vi "MassData Parameter Support Demo.vi"() -> ()   [LabVIEW 2017]
uses:
  MassData-Parameter/_support/Operation-FGV-MassData.ctl
  b1bc9acf-e850-46c1-b3cf-cc66e9187574.vi
  537af5e7-dcec-4c12-9422-676432e19088.vi
  MassData-Parameter/CSM MassData Parameter Support.lvlib
panel:
  in  "stop":bool
  out "Thermometer":cluster{dbl, dbl}(slide)={0.0, 6224.489795918367} scale=0.0..1000000.0 scale format="%#_6p"
  out "Argument":string
  out "Waveform Graph":i32[](graph)
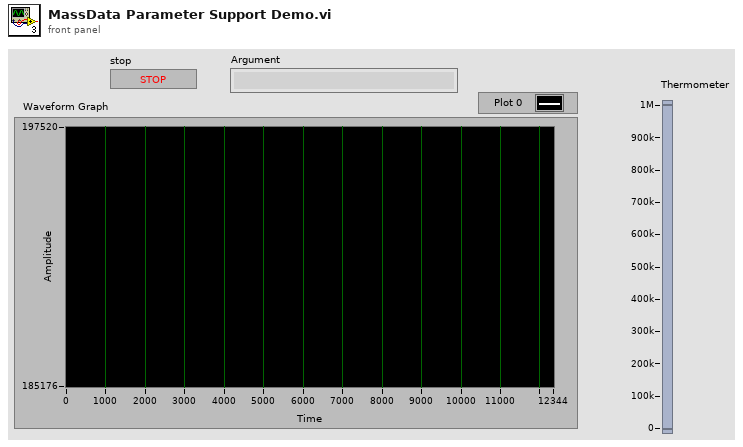
[diagram p1: front panel]
types:
  T1 = typedef "CSM MassData Parameter Support.lvlib/Operation-FGV-MassData.ctl" = enum16{"Initialize", "Read", "Write", "Status", "Release"}
  T2 = typedef "CSM MassData Parameter Support.lvlib/Def-MassDataOper-Status.ctl" = cluster{"Start":i32, "Size":i32, "Total":i32}
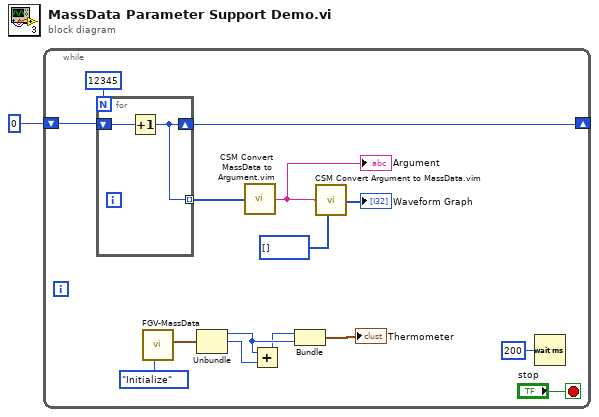
[diagram p0: block diagram]
diagram:
  n1 = while {
    shift-right: [w4] -> _
    shift-left: 0 -> [w5]
    stop <- "stop" stop-if-true
    n2 = for {
      N: 12345 -> [_]
      tunnel: [w17] -> w15 mode=indexing
      shift-right: [w17] -> w4
      shift-left: w5 -> [w18]
      n3 = Increment(x=w18) -> (x+1=w17:i32)
    }
    n4 = call "FGV-MassData.vi"("Operation"=Operation-FGV-MassData."Initialize") -> ("Active Write Oper"=w8:T2)  [unwired: 7 in, 3 out]
    n5 = Unbundle(w8) -> ("Start"=w11:i32, "Size"=w9:i32)  [unwired: 1 out]
    n6 = call "CSM Convert MassData to Argument.vim"("DBL"=w15) -> ("Argument"=w2:string)  [unwired: 8 in]
    "Argument" <- w2
    n7 = Add(x=w11, y=w9) -> (x+y=w10:i32)
    n8 = Bundle(w10, "Start"=w11) -> (→"Thermometer":cluster{i32, "Start":i32})  [unwired: 1 in]
    n9 = call "CSM Convert Argument to MassData.vim"("Type"=i32[] [], "HEX Argument"=w2) -> ("DBL"=→"Waveform Graph":i32[])  [unwired: 7 in]
    n10 = Wait (ms)(milliseconds to wait=u32 200) -> ()  [unwired: 1 out]
  }
